vi "setup_lc_gh.vi"(6 "yw":string, 7 "zc_luodi_num":string, 8 "didian":string, 9 "shuoming":string, 10 "id":string, 11 "jsren":string) -> (0 "error":errorcluster caption="error out 2")   [LabVIEW 2017, in "Lib_code.lvlib"]
uses:
  Lib_code.lvlib
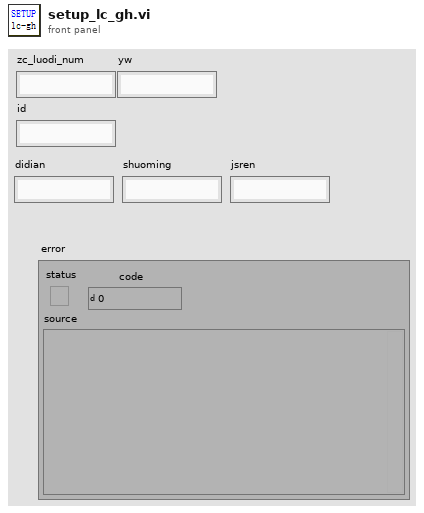
[diagram p1: front panel]
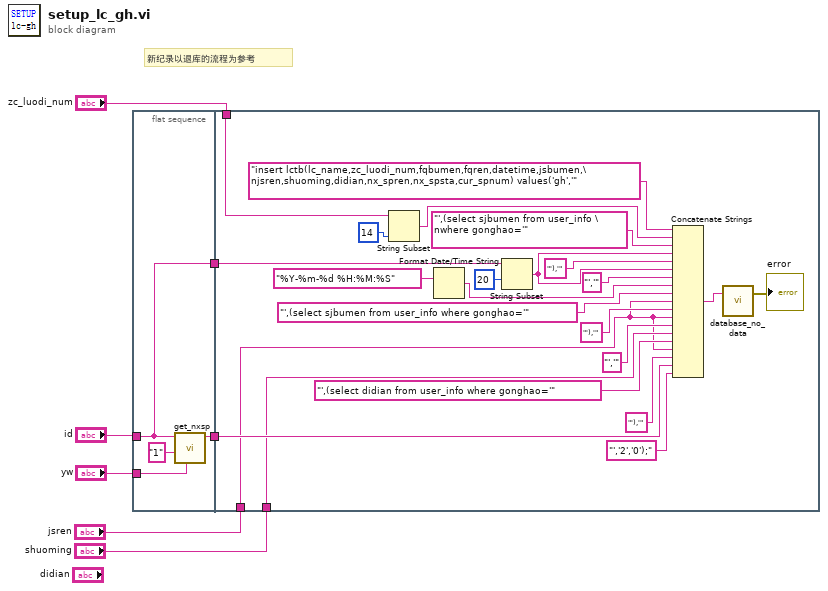
[diagram p0: block diagram]
diagram:
  # "新纪录以退库的流程为参考"
  n1 = flat-sequence {
    tunnel: [w11] -> w7
    tunnel: [w10] -> w6
    tunnel: "id" -> [w10]
    tunnel: "yw" -> [w9]
    tunnel: w7 -> [w26]
    tunnel: w6 -> [w18]
    tunnel: "shuoming" -> [w19]
    tunnel: "zc_luodi_num" -> [w23]
    tunnel: "jsren" -> [w12]
    frame #0 {
      n2 = call "get_nxsp.vi"("yw"=w9, "Cur_state"="1", "fqren"=w10) -> ("sp_gonghao"=w11:string)  [unwired: 6 in, 2 out]
    }
    frame #1 {
      n3 = String Subset(string=w23, length (rest)=14 ("长度（剩余）")) -> (substring=w31:string)  [unwired: 1 in]
      n4 = Format Date/Time String(time format string (%c)="%Y-%m-%d %H:%M:%S" ("时间格式字符串(%c)")) -> (date/time string=w15:string)  [unwired: 2 in]
      n5 = String Subset(string=w18, length (rest)=20 ("长度（剩余）")) -> (substring=w17:string)  [unwired: 1 in]
      n6 = Concatenate Strings("insert lctb(lc_name,zc_luodi_num,fqbumen,fqren,datetime,jsbumen,\njsren,shuoming,didian,nx_spren,nx_spsta,cur_spnum) values('gh','" ("格式字符串"), w31, "',(select sjbumen from user_info \nwhere gonghao='" ("字符串"), w17, "'),'" ("字符串"), w17, "','" ("字符串"), w15, "',(select sjbumen from user_info where gonghao='" ("字符串"), w12, "'),'" ("字符串"), w12, "','" ("字符串"), w19, "',(select didian from user_info where gonghao='" ("字符串"), w12, "'),'" ("字符串"), w26, "','2','0');" ("字符串")) -> (w22:string)
      n7 = call "database_no_data.vi"("input"=w22) -> ("error"=→"error":errorcluster)  [unwired: 2 in]
    }
  }
